vi "pixy pid.vi"() -> ()   [LabVIEW 2019]
uses:
  <vilib>/addons/control/pid/NI_PID_pid.lvlib
  <instrlib>/Charmed Labs/Pixy2/library/Types/Block.ctl
  <instrlib>/Charmed Labs/Pixy2/library/Pixy2.lvlib
  <vilib>/addons/control/pid/pid.llb/PID (DBL).vi
panel:
  in  "PID gains forward velocity":T1={"proportional gain (Kc)"=1.0, "integral time (Ti, min)"=0.01, "derivative time (Td, min)"=0.0} {"derivative time (Td, min)" format="%.3f"; "integral time (Ti, min)" format="%.3f"; "proportional gain (Kc)" format="%.3f"}
  in  "area set point":dbl
  out "right":dbl
  out "left":dbl
  in  "blocks":T2[](array[typedef])
  in  "PID gains rotation":T1={"proportional gain (Kc)"=1.0, "integral time (Ti, min)"=0.01, "derivative time (Td, min)"=0.0} {"derivative time (Td, min)" format="%.3f"; "integral time (Ti, min)" format="%.3f"; "proportional gain (Kc)" format="%.3f"}
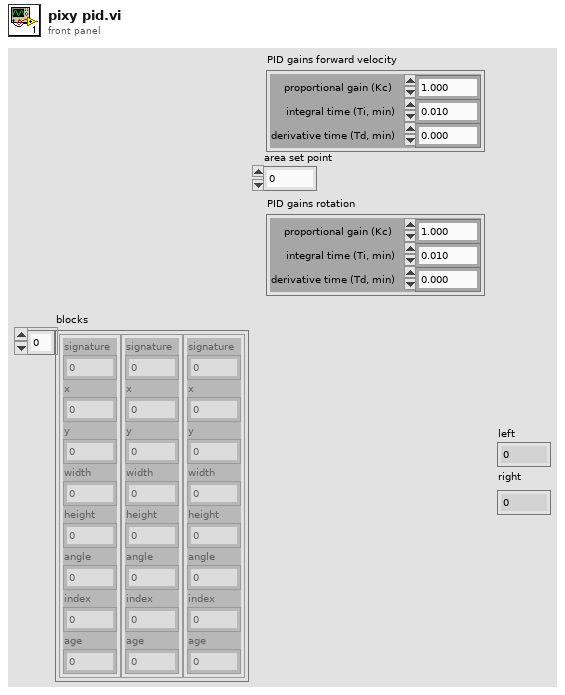
[diagram p1: front panel]
types:
  T1 = cluster{"proportional gain (Kc)":dbl, "integral time (Ti, min)":dbl, "derivative time (Td, min)":dbl}
  T2 = typedef "Pixy2.lvlib/Block.ctl" = cluster{"signature":u16, "x":u16, "y":u16, "width":u16, "height":u16, "angle":i16, "index":u8, "age":u8}
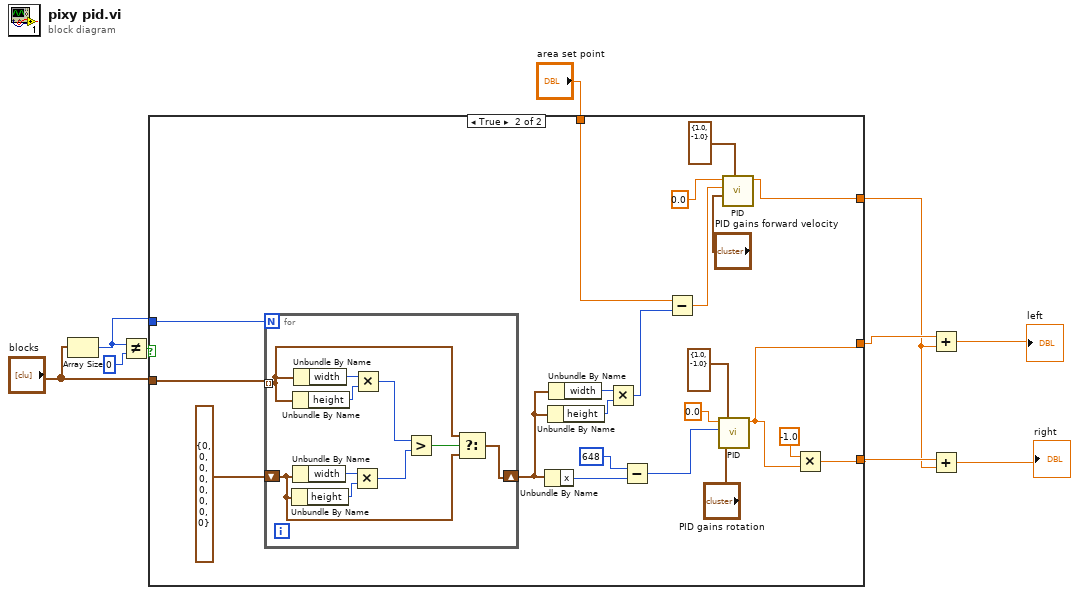
[diagram p0: block diagram]
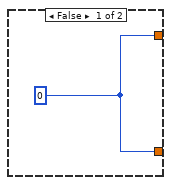
[diagram p2: hidden frame]
diagram:
  n1 = Array Size(array="blocks") -> (size(s)=w8:i32)
  n2 = Not Equal?(x=w8, y=0) -> (x != y?=w10:bool)
  n3 = case shown="True" w10 {
    tunnel: "blocks" -> [_ w33]
    tunnel: w8 -> [_ w32]
    tunnel: [w11 w27] -> w4
    tunnel: [w11 w26] -> w5
    tunnel: "area set point" -> [_ w13]
    tunnel: [_ w14] -> w3
    frame False {
      w11 = 0
    }
    frame True {
      n4 = for {
        N: w32 -> [_]
        tunnel: w33 -> [w37] mode=indexing
        shift-right: [w35] -> w19
        shift-left: T2 {"signature"=0, "x"=0, "y"=0, "width"=0, "height"=0, "angle"=0, "index"=0, "age"=0} ("block") -> [w36]
        n5 = Unbundle By Name(w36) -> ("height"=w40:u16)
        n6 = Unbundle By Name(w37) -> ("height"=w42:u16)
        n7 = Unbundle By Name(w36) -> ("width"=w39:u16)
        n8 = Unbundle By Name(w37) -> ("width"=w43:u16)
        n9 = Multiply(x=w39, y=w40) -> (x*y=w38:u16)
        n10 = Multiply(x=w43, y=w42) -> (x*y=w34:u16)
        n11 = Greater?(x=w34, y=w38) -> (0:w41:bool)
        n12 = Select(t=w37, s=w41, f=w36) -> (s? t:f=w35:T2)
      }
      n13 = Unbundle By Name(w19) -> ("x"=w24:u16)
      n14 = Unbundle By Name(w19) -> ("height"=w20:u16)
      n15 = Unbundle By Name(w19) -> ("width"=w21:u16)
      n16 = Multiply(x=w21, y=w20) -> (x*y=w12:u16)
      n17 = Subtract(x=648 ("index"), y=w24) -> (x-y=w22:i32)
      n18 = Subtract(x=w13, y=w12) -> (x-y=w15:dbl)
      n19 = call-poly <vilib>:"PID.vi"("output range"=cluster{"output high":dbl, "output low":dbl} {"output high"=1.0, "output low"=-1.0}, "PID gains"="PID gains rotation", "process variable"=w22, "setpoint"=0.0) -> ("output"=w27:dbl)  [unwired: 6 in, 1 out]
      n20 = call-poly <vilib>:"PID.vi"("output range"=cluster{"output high":dbl, "output low":dbl} {"output high"=1.0, "output low"=-1.0}, "PID gains"="PID gains forward velocity", "process variable"=w15, "setpoint"=0.0) -> ("output"=w14:dbl)  [unwired: 6 in, 1 out]
      n21 = Multiply(x=-1.0, y=w27) -> (x*y=w26:dbl)
    }
  }
  n22 = Add(x=w4, y=w3) -> (x+y=→"left":dbl)
  n23 = Add(x=w5, y=w3) -> (x+y=→"right":dbl)
